vi "Destroy.vi"(7 "Actor in":refnum<class "Actor.lvclass">, 11 "Msg State in":refnum<class "Msg State.lvclass">) -> (5 "Actor out":refnum<class "Actor.lvclass">)   [LabVIEW 2021, in "jettl.lvlib" / "Msg State.lvclass"]
uses:
  Msg State.lvclass
  Actor/Actor/Actor.lvclass
  Actor/Msgs/Destroy/Destroy Msg/Destroy Msg.lvclass
  C:/git/jettl/src/Actor/Msg/Msg.lvclass
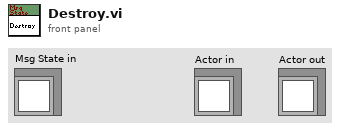
[diagram p1: front panel]
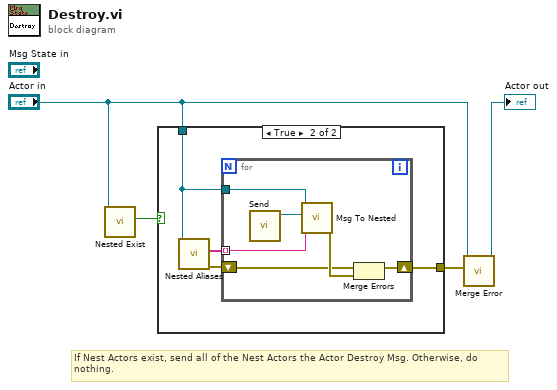
[diagram p0: block diagram]
diagram:
  # "If Nest Actors exist, send all of the Nest Actors the Actor Destroy Msg. Otherwise, do nothing."
  n1 = call-dynamic "Nested Exist.vi"("Actor in"="Actor in") -> ("Nested Exist?"=w4:bool)  [unwired: 10 in]
  n2 = case shown="True" w4 {
    tunnel: [_ w8] -> w2
    tunnel: "Actor in" -> [_ w5]
    frame False {
    }
    frame True {
      n3 = call-dynamic "Nested Aliases.vi"("Actor in"=w5) -> ("error out"=w6:errorcluster, "Nested Aliases"=w7:string[])  [unwired: 9 in]
      n4 = for {
        tunnel: w7 -> [w11] mode=indexing
        shift-right: [w14] -> w8
        shift-left: w6 -> [w9]
        tunnel: w5 -> [w13]
        n5 = call "Send.vi"() -> ("Destroy Msg out"=w12:refnum<class "Destroy Msg.lvclass">)  [unwired: 11 in]
        n6 = call-dynamic "Msg To Nested.vi"("Alias"=w11, "Msg"=w12, "Actor in"=w13) -> ("error out"=w10:errorcluster)  [unwired: 8 in]
        n7 = Merge Errors(w9, w10) -> (w14:errorcluster)
      }
    }
  }
  n8 = call-dynamic "Merge Error.vi"("Error"=w2, "Set Error in"="Actor in") -> ("Set Error out"=→"Actor out":refnum<class "Actor.lvclass">)  [unwired: 9 in]
